vi "Clear Light State.vi"(8 "error in":errorcluster, 11 "Light Stack in":refnum<class "Light Stack.lvclass">) -> (0 "error out":errorcluster, 3 "Light Stack out":refnum<class "Light Stack.lvclass">)   [LabVIEW 2018, in "Light Stack.lvlib" / "Light Stack.lvclass"]
uses:
  Light Stack.lvclass
  Light Stack.lvclass/Light Stack.ctl
  Custom Controls/Light Mode.ctl
  Light Stack.lvlib
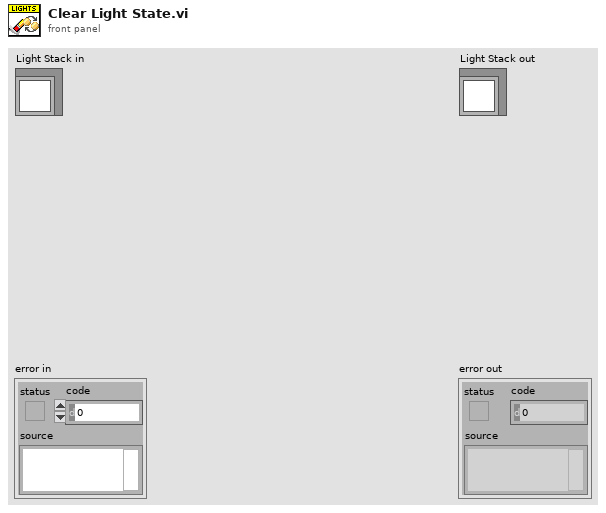
[diagram p1: front panel]
types:
  T1 = typedef "Light Stack.lvlib/Light Mode.ctl" = enum16{"OFF", "ON", "BLINK"}
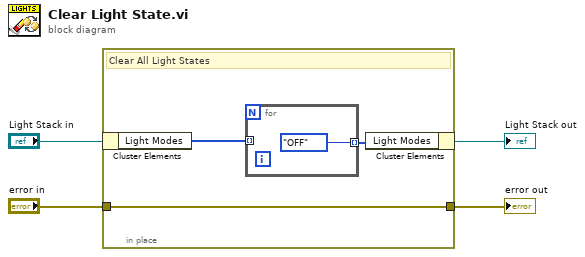
[diagram p0: block diagram]
diagram:
  n1 = in-place {
    in-place-border: "error in" -> [w5]
    in-place-border: [w5] -> w1
    # "Clear All Light States"
    n2 = in-place-cluster #1("Light Stack in") -> ("Light Modes"=w7:T1[])
    n3 = for {
      tunnel: w7 -> [_] mode=indexing
      tunnel: [Light_Mode."OFF" ("State")] -> w6 mode=indexing
    }
    n4 = in-place-cluster #1("Light Modes"=w6) -> (→"Light Stack out":refnum<class "Light Stack.lvclass">)
  }
  "error out" <- w1
